vi "PCE_ANSWER.vi"(0 "Commande\neffectuée ?":bool, 1 "VISA resource name":refnum<visa-resource-name>) -> ()   [LabVIEW 2010]
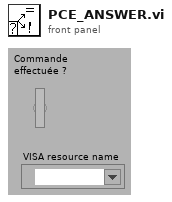
[diagram p1: front panel]
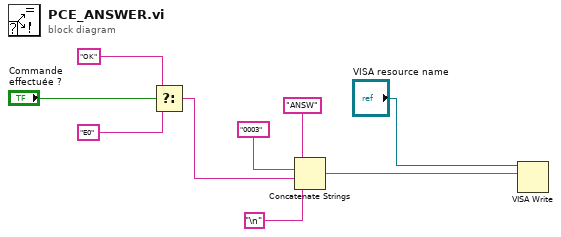
[diagram p0: block diagram]
diagram:
  n1 = Select(t="OK", s="Commande\neffectuée ?", f="E0") -> (s? t:f=w5:string)
  n2 = Concatenate Strings("ANSW", "0003" ("élément"), w5, "\n" ("élément")) -> (w1:string)
  n3 = VISA Write(VISA resource name="VISA resource name", write buffer=w1) -> ()  [unwired: 1 in, 3 out]
